vi "Butterworth_zerophase_filter.vi"(6 "order":i32=2, 7 "filter type":T1, 8 "low cutoff freq: fl":dbl=0.12500000000000006 format="%0.4f", 9 "high cutoff freq: fh":dbl=0.45000000000000007 format="%0.2f", 10 "sampling freq: fs":dbl=1.0 format="%0.2f", 11 "X":dbl[](array[numeric])) -> (1 "error":i32, 3 "Filtered X":dbl[](array[numeric]))   [LabVIEW 2016]
uses:
  <vilib>/Analysis/3filter.llb/Filter Passband Type.ctl
  <vilib>/Analysis/3filter.llb/Zero Phase Filter (DBL).vi
  <vilib>/Analysis/NI_AALBase.lvlib
panel:
  in  "?":dbl[](array[numeric]) format="%0.2f"
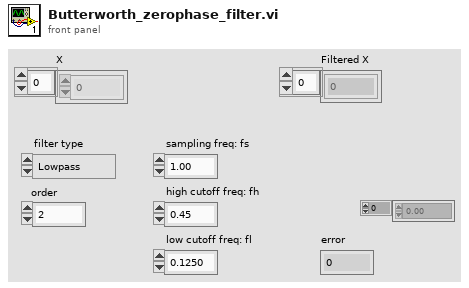
[diagram p1: front panel]
types:
  T1 = typedef "NI_AALBase.lvlib/Filter Passband Type.ctl" = enum32{"Lowpass", "Highpass", "Bandpass", "Bandstop"}
  T2 = cluster{"filter structure":enum32{"IIR 2nd Order", "IIR 4th Order"}, "Reverse Coefficients":dbl[], "Forward Coefficients":dbl[]}
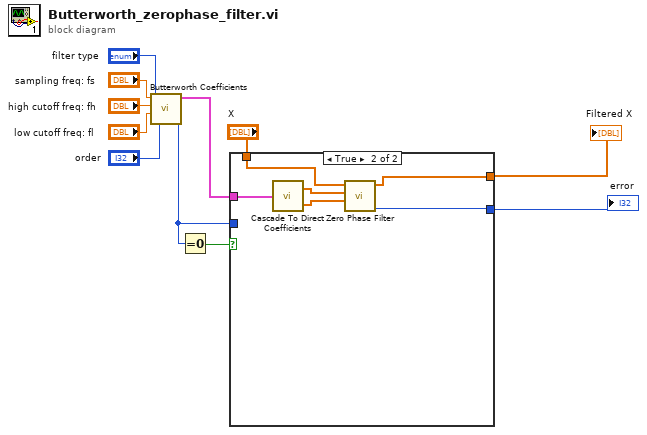
[diagram p0: block diagram]
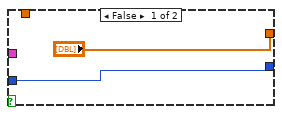
[diagram p2: hidden frame]
diagram:
  n1 = call <vilib>:"Butterworth Coefficients.vi"("order"="order", "filter type"="filter type", "low cutoff freq: fl"="low cutoff freq: fl", "high cutoff freq: fh"="high cutoff freq: fh", "sampling freq: fs"="sampling freq: fs") -> ("error"=w2:i32, "IIR Filter Cluster"=w4:T2)  [unwired: 5 in]
  n2 = Equal To 0?(x=w2) -> (x = 0?=w3:bool)
  n3 = case shown="True" w3 {
    tunnel: w2 -> [w13 _]
    tunnel: "X" -> [_ w16]
    tunnel: ["?" w15] -> w10
    tunnel: w4 -> [_ w19]
    tunnel: [w13 w14] -> w9
    frame False {
    }
    frame True {
      n4 = call <vilib>:"Cascade To Direct Coefficients.vi"("IIR Filter Cluster"=w19) -> ("Reverse Coefficients"=w18:dbl[], "Forward Coefficients"=w17:dbl[])
      n5 = call-poly <vilib>:"Zero Phase Filter.vi"("Forward Coefficients"=w17, "Reverse Coefficients"=w18, "X"=w16) -> ("error"=w14:i32, "Filtered X"=w15:dbl[])  [unwired: 7 in]
    }
  }
  "Filtered X" <- w10
  "error" <- w9
